vi "Initialize Error Log File.vi"(8 "Error In":errorcluster, 11 "Error Handling In":refnum<class "Error Handling.lvclass">) -> (0 "Error Out":errorcluster, 3 "Error Handling Out":refnum<class "Error Handling.lvclass">)   [LabVIEW 2019, in "Error Handling.lvclass"]
uses:
  Error Handling.lvclass
  Accessors/Log File Reference/Set Log File Reference.vi
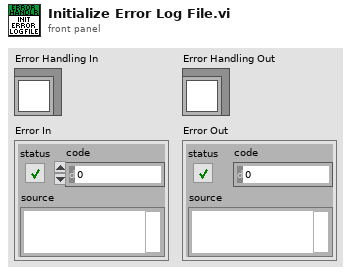
[diagram p1: front panel]
types:
  T1 = enum16{"open", "replace", "create", "open or create", "replace or create", "replace or create with confirmation"}
  T2 = typedef "LVDateTimeRec.ctl" = cluster{"fractional second":dbl, "second":i32, "minute":i32, "hour":i32, "day of month":i32, "month":i32, "year":i32, "day of week":i32, "day of year":i32, "DST":i32}
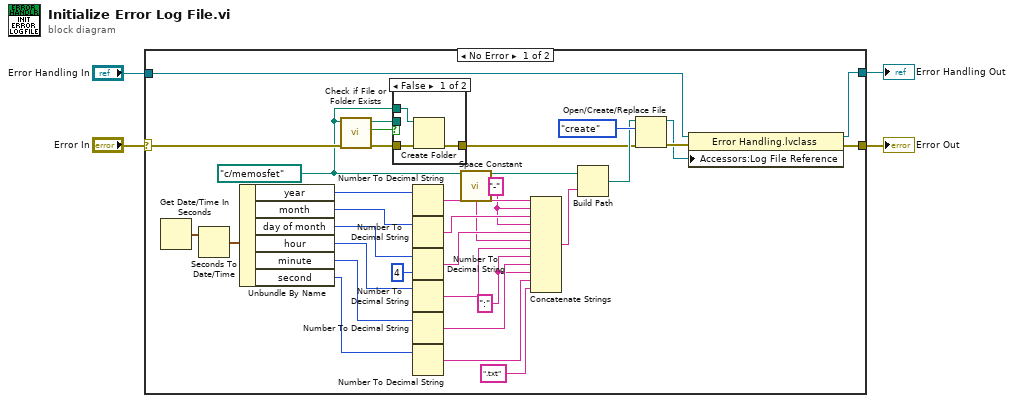
[diagram p0: block diagram]
diagram:
  n1 = case shown="No Error" "Error In" {
    selector: "Error In" -> [w13 w42]
    tunnel: "Error Handling In" -> [w35 w43]
    tunnel: [w34 w43] -> w2
    tunnel: [w33 w42] -> w1
    frame No Error {
      w7 = ":"
      w19 = "-"
      w10 = path "c:/memosfet" ("file path (use dialog)")
      n2 = Get Date/Time In Seconds() -> (seconds since 1Jan1904=w30:timestamp)
      n3 = Seconds To Date/Time(time stamp (now)=w30) -> (date time rec=w29:T2)  [unwired: 1 in]
      n4 = Unbundle By Name(w29) -> ("year"=w27:i32, "month"=w26:i32, "day of month"=w25:i32, "hour"=w24:i32, "minute"=w23:i32, "second"=w6:i32)
      n5 = call <vilib>:"Check if File or Folder Exists.vi"("error in (no error)"=w13, "path"=w10) -> ("error out"=w12:errorcluster, "file or folder exists?"=w11:bool, "dup path"=w8:path)  [unwired: 7 in]
      n6 = case shown="False" w11 {
        tunnel: w12 -> [w39 w41]
        tunnel: w10 -> [w40 _]
        tunnel: [w38 w41] -> w9
        tunnel: w8 -> [_ _]
        frame False {
          n7 = Create Folder(path (use dialog)=w40, error in=w39) -> (error out=w38:errorcluster)  [unwired: 1 in, 2 out]
        }
        frame True {
        }
      }
      n8 = Number To Decimal String(number=w27) -> (decimal integer string=w21:string)  [unwired: 1 in]
      n9 = Number To Decimal String(number=w26) -> (decimal integer string=w20:string)  [unwired: 1 in]
      n10 = Number To Decimal String(number=w25, width (-)=i16 4) -> (decimal integer string=w18:string)
      n11 = Number To Decimal String(number=w24) -> (decimal integer string=w16:string)  [unwired: 1 in]
      n12 = Number To Decimal String(number=w23) -> (decimal integer string=w15:string)  [unwired: 1 in]
      n13 = Number To Decimal String(number=w6) -> (decimal integer string=w5:string)  [unwired: 1 in]
      n14 = call <vilib>:"Space Constant.vi"() -> ("String"=w17:string)
      n15 = Concatenate Strings(w21, w19, w20, w19, w18, w17, w16, w7, w15, w7, w5, ".txt" ("string")) -> (w28:string)
      n16 = Build Path(base path=w10, name or relative path=w28) -> (appended path=w32:path)
      n17 = Open/Create/Replace File(file path (use dialog)=w32, error in=w9, operation (0:open)=T1."create") -> (refnum out=w31:refnum<file>, error out=w37:errorcluster)  [unwired: 3 in, 1 out]
      n18 = property class="Error Handling.lvclass"(reference=w35, error in=w37, "Accessors:Log File Reference"=w31) -> (reference out=w34:refnum<class "Error Handling.lvclass">, error out=w33:errorcluster)
    }
    frame Error {
    }
  }
  "Error Handling Out" <- w2
  "Error Out" <- w1
